vi "lib SCLK to LV Timestamp.vi"(8 "error in (no error)":errorcluster, 11 "SCLK":dbl format="%#_11f") -> (0 "error out":errorcluster, 3 "lv timestamp":timestamp format="%<%H:%M:%S%3u\n%x>T")   [LabVIEW 2011]
panel:
  in  "J2000 Epoch":timestamp=timestamp(3029590736 s since 1904-01-01) format="%<%H:%M:%S%2u\n%x>T"
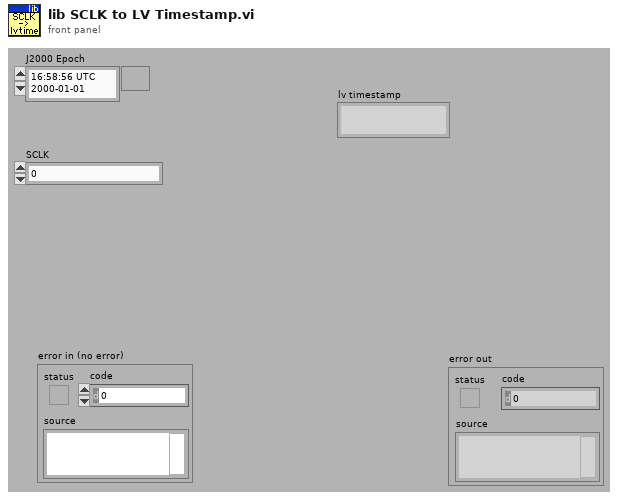
[diagram p1: front panel]
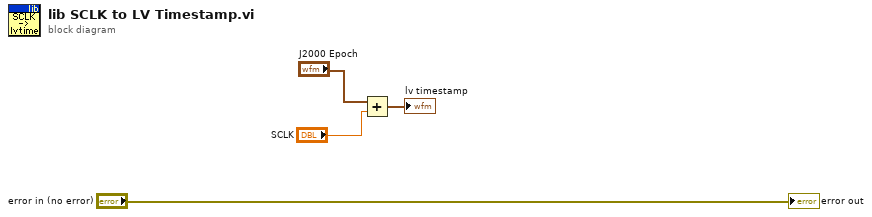
[diagram p0: block diagram]
diagram:
  n1 = Add(x="J2000 Epoch", y="SCLK") -> (x+y=→"lv timestamp":timestamp)
  "error out" <- "error in (no error)"
